vi "Actor Core.vi"(8 "error in":errorcluster, 11 "Sine in":refnum<class "Rigol DG822 Sine.lvclass">) -> (0 "error out":errorcluster, 3 "Actor out":refnum<class "Actor.lvclass">)   [LabVIEW 2021, in "Rigol DG822 UI.lvlib" / "Rigol DG822 Sine.lvlib" / "Rigol DG822 Sine.lvclass"]
uses:
  Rigol DG822 Sine.lvclass
  D:/LabVIEW/General/Files/lvlibp/Actors.lvlibp/Actors/Actors/Actors.lvclass
  General/Files/lvlibp/Actor Framework.lvlibp/1abvi3w/vi.lib/ActorFramework/Actor/Actor.lvclass
  Rigol DG822 UI/lib/controls.llb/WaveformParamTags.ctl
  Rigol DG822 UI/lib/controls.llb/FreqUnitHandler.ctl
  Rigol DG822 UI/lib/controls.llb/DataCluster.ctl
  Rigol DG822 UI/lib/controls.llb/PeriodUnitHandler.ctl
  Rigol DG822 UI/lib/controls.llb/AmplUnitHandler.ctl
  Rigol DG822 UI/lib/controls.llb/HighLUnitHandler.ctl
  Rigol DG822 UI/lib/controls.llb/OffsetUnitHandler.ctl
  Rigol DG822 UI/lib/controls.llb/LowLUnitHandler.ctl
  Rigol DG822 UI/lib/controls.llb/PhaseUnitHandler.ctl
  Rigol DG822 UI/lib/controls.llb/FreqUnit.ctl
  Rigol DG822 UI/lib/controls.llb/PeriodUnit.ctl
  Rigol DG822 UI/lib/controls.llb/AmplUnit.ctl
  Rigol DG822 UI/lib/controls.llb/HighLUnit.ctl
  Rigol DG822 UI/lib/controls.llb/OffsetUnit.ctl
  Rigol DG822 UI/lib/controls.llb/LowLUnit.ctl
  Rigol DG822 UI/lib/controls.llb/SineParamDisplay.ctl
  Rigol DG822 UI/lib/controls.llb/StringIndicatorSelected.ctl
  Rigol DG822 UI/lib/controls.llb/RDG822ExtCall.ctl
  Rigol DG822 UI/lib/controls.llb/FT Controls Cluster.ctl
  Rigol DG822 Sine.lvclass/Rigol DG822 Sine.ctl
  Rigol DG822 UI/lib/controls.llb/WaveformExtCall.ctl
  Rigol DG822 UI/lib/controls.llb/AllWaveformDataCluster.ctl
  Rigol DG822 UI/lib/controls.llb/String Indicators Cluster.ctl
  <vilib>/Utility/miscctls.llb/LVPointTypeDef.ctl
  <userlib>/_MGI/Application Control/MGI VI Reference/MGI Current VI's Reference.vi
  General/Files/lvlibp/Actors.lvlibp/Actors/Actors/Actors.lvclass
panel:
  in  "ParamTags":T1
  out "Data":T2={"Freq"={"Freq"=1.0, "FreqUnit"=enum."kHz", "FreqUnitPrcs"=9.0}, "Period"={"Period"=1.0, "PeriodUnit"=enum."ms", "PeriodUnitPrcs"=7.0}, "Ampl"={"Ampl"=5.0, "AmplUnit"=enum."Vpp", "AmplUnitPrcs"=4.0}, "HighL"={"HighL"=2.5, "HighLUnit"=enum."V", "HighLUnitPrcs"=4.0}, "Offset"={"Offset"=0.0, "OffsetUnit"=enum."Vdc", "OffsetUnitPrcs"=4.0}, "LowL"={"LowL"=-2.5, "LowLUnit"=enum."V", "LowLUnitPrcs"=4.0}, "Phase"={"Phase"=0.0, "PhaseUnit"=enum."°", "PhaseUnitPrcs"=3.0}, "Duty"={"Duty"=50.0, "DutyUnit"=enum."%", "DutyUnitPrcs"=3.0}, "Width"={"Width"=500.0, "WidthUnit"=enum."us", "WidthUnitPrcs"=4.0}, "RisEdge"={"RisEdge"=10.0, "RisEdgeUnit"=enum."ns", "RisEdgeUnitPrcs"=1.0}, "FallEdge"={"FallEdge"=10.0, "FallEdgeUnit"=enum."ns", "FallEdgeUnitPrcs"=1.0}} {"RisEdge"."RisEdge" format="%.1f"; "RisEdge"."RisEdgeUnitPrcs" format="%#_1g"; "FallEdge"."FallEdge" format="%.1f"; "FallEdge"."FallEdgeUnitPrcs" format="%#_1g"; "Width"."Width" format="%.4g"; "Width"."WidthUnitPrcs" format="%#_1g"; "Duty"."Duty" format="%.3g"; "Duty"."DutyUnitPrcs" format="%#_1g"; "Phase"."Phase" format="%.3g"; "Phase"."PhaseUnitPrcs" format="%#_1g"; "LowL"."LowL" format="%.4g"; "LowL"."LowLUnitPrcs" format="%#_1g"; "Offset"."Offset" format="%.4g"; "Offset"."OffsetUnitPrcs" format="%#_1g"; "HighL"."HighL" format="%.4g"; "HighL"."HighLUnitPrcs" format="%#_1g"; "Ampl"."Ampl" format="%.4g"; "Ampl"."AmplUnitPrcs" format="%#_1g"; "Period"."Period" format="%.7g"; "Period"."PeriodUnitPrcs" format="%#_1g"; "Freq"."FreqUnitPrcs" format="%#_1g"; "Freq"."Freq" format="%.9g"}
  in  "Conf Tabs":enum32{"Sine", "OK"}(tab)
  out "SineParamDisplay":T3
  out "String Indcs":T4={"Freq-Period"="1.000,000,000 kHz", "Ampl-HighL"="5.000,0 Vpp", "Offset-LowL"="0.000,0 Vdc", "Phase"="0.000 °"}
  in  "F/T Ctrls":T5
  in  "Value":dbl=1.0 format="%.8g"
  in  "Unit Tabs":T6(tab)
  out "FreqUnitHandler":T7=1
  in  "FreqUnit":T8=enum."kHz"
  out "PeriodUnitHandler":T9=1
  in  "PeriodUnit":T10=enum."ms"
  in  "AmplUnit":T11=enum."Vpp"
  out "AmplUnitHandler":T12
  out "HighLUnitHandler":T13
  in  "HighLUnit":T14=enum."V"
  out "OffsetUnitHandler":T15
  in  "OffsetUnit":T16=enum."Vdc"
  out "LowLUnitHandler":T17
  in  "LowLUnit":T18=enum."V"
  out "PhaseUnitHandler":T19
  in  "OK":bool
  # "MHz - 10 \nkHz - 9\nHz - 6\nmHz - 3\nuHz - 0?"
  # "s - 10\nms - 7\nus - 4 \nns - 1?"
  # "All 4 - V - 4\n        mV - 1"
  # "no change"
  # "no change"
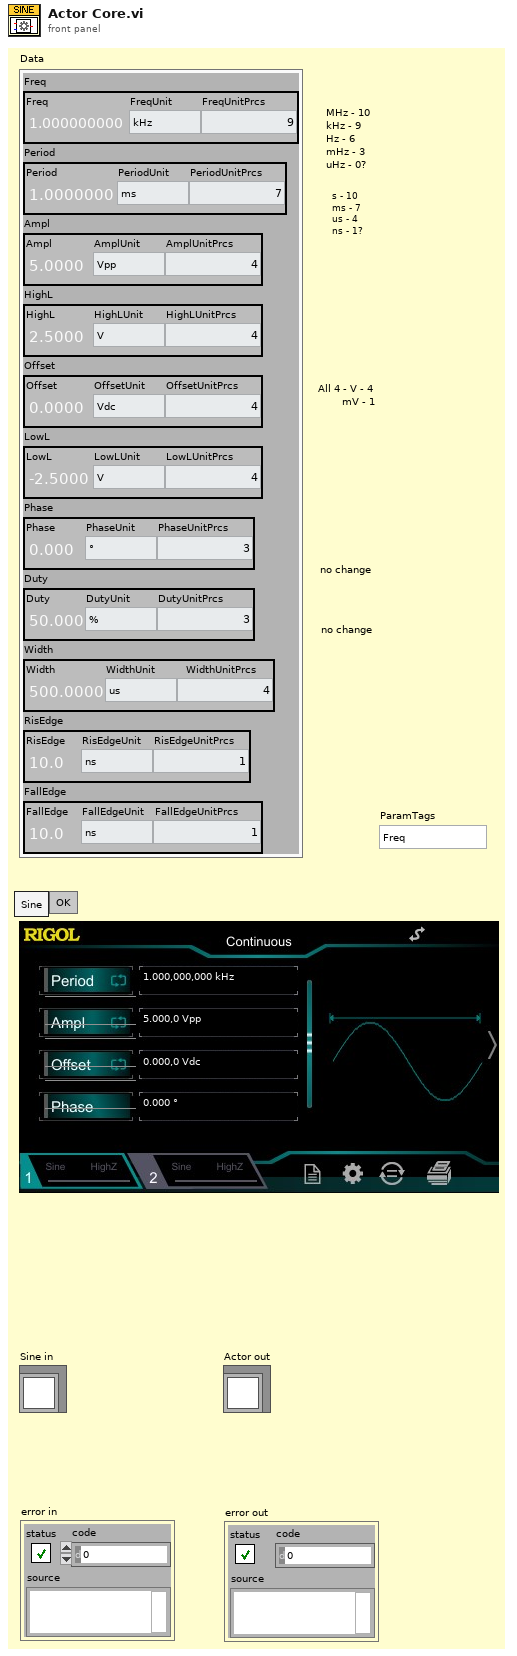
[diagram p1: front panel]
types:
  T1 = typedef "WaveformParamTags.ctl" = enum16{"Freq", "Period", "Ampl", "HighL", "Offset", "LowL", "Phase", "Duty", "Width", "RisEdge", "FallEdge"}
  T2 = typedef "DataCluster.ctl" = cluster{"Freq":cluster{"Freq":dbl, "FreqUnit":enum32{"No Selection", "MHz", "kHz", "Hz", "mHz", "uHz"}, "FreqUnitPrcs":dbl}, "Period":cluster{"Period":dbl, "PeriodUnit":enum32{"No Selection", "s", "ms", "us", "ns"}, "PeriodUnitPrcs":dbl}, "Ampl":cluster{"Ampl":dbl, "AmplUnit":enum32{"No Selection", "Vpp", "mVpp"}, "AmplUnitPrcs":dbl}, "HighL":cluster{"HighL":dbl, "HighLUnit":enum32{"No Selection", "V", "mV"}, "HighLUnitPrcs":dbl}, "Offset":cluster{"Offset":dbl, "OffsetUnit":enum32{"No Selection", "Vdc", "mVdc"}, "OffsetUnitPrcs":dbl}, "LowL":cluster{"LowL":dbl, "LowLUnit":enum32{"No Selection", "V", "mV"}, "LowLUnitPrcs":dbl}, "Phase":cluster{"Phase":dbl, "PhaseUnit":enum32{"°"}, "PhaseUnitPrcs":dbl}, "Duty":cluster{"Duty":dbl, "DutyUnit":enum32{"%"}, "DutyUnitPrcs":dbl}, "Width":cluster{"Width":dbl, "WidthUnit":enum32{"No Selection", "s", "ms", "us", "ns"}, "WidthUnitPrcs":dbl}, "RisEdge":cluster{"RisEdge":dbl, "RisEdgeUnit":enum32{"No Selection", "s", "ms", "us", "ns"}, "RisEdgeUnitPrcs":dbl}, "FallEdge":cluster{"FallEdge":dbl, "FallEdgeUnit":enum32{"No Selection", "s", "ms", "us", "ns"}, "FallEdgeUnitPrcs":dbl}}
  T3 = typedef "SineParamDisplay.ctl" = u16
  T4 = cluster{"Freq-Period":string, "Ampl-HighL":string, "Offset-LowL":string, "Phase":string}
  T5 = cluster{"Freq/Period":bool, "Ampl/HighL":bool, "Offset/LowL":bool}
  T6 = enum32{"Freq", "Period", "Ampl", "HighL", "Offset", "LowL", "Phase"}
  T7 = typedef "FreqUnitHandler.ctl" = u16
  T8 = typedef "FreqUnit.ctl" = enum32{"No Selection", "MHz", "kHz", "Hz", "mHz", "uHz"}
  T9 = typedef "PeriodUnitHandler.ctl" = u16
  T10 = typedef "PeriodUnit.ctl" = enum32{"No Selection", "s", "ms", "us", "ns"}
  T11 = typedef "AmplUnit.ctl" = enum32{"No Selection", "Vpp", "mVpp"}
  T12 = typedef "AmplUnitHandler.ctl" = u16
  T13 = typedef "HighLUnitHandler.ctl" = u16
  T14 = typedef "HighLUnit.ctl" = enum32{"No Selection", "V", "mV"}
  T15 = typedef "OffsetUnitHandler.ctl" = u16
  T16 = typedef "OffsetUnit.ctl" = enum32{"No Selection", "Vdc", "mVdc"}
  T17 = typedef "LowLUnitHandler.ctl" = u16
  T18 = typedef "LowLUnit.ctl" = enum32{"No Selection", "V", "mV"}
  T19 = typedef "PhaseUnitHandler.ctl" = u16
  T20 = cluster{"Freq-Period":string, "Freq-Period 2":string, "Freq-Period 3":string, "Freq-Period 4":string}
  T21 = typedef "LVPointTypeDef.ctl" = cluster{"Horizontal":i16, "Vertical":i16}
  T22 = typedef "StringIndicatorSelected.ctl" = enum16{"Freq-Period", "Ampl-HighL", "Offset-LowL", "Phase", "Duty-Width", "RisEdge", "FallEdge"}
  T23 = typedef "FT Controls Cluster.ctl" = cluster{"Freq/Period":bool, "Ampl/HighL":bool, "Offset/LowL":bool, "Duty/Width":bool}
  T24 = typedef "RDG822ExtCall.ctl" = enum16{"Get Data"}
  T25 = typedef "WaveformExtCall.ctl" = enum16{"Freq", "Period", "Ampl", "HighL", "Offset", "LowL", "Phase", "Duty", "Width", "RisEdge", "FallEdge", "Home", "InitData"}
  T26 = cluster{"Freq":cluster{"Freq":dbl, "FreqUnit":enum32{"No Selection", "MHz", "kHz", "Hz", "mHz", "uHz"}, "FreqUnitPrcs":dbl}, "Period":cluster{"Period":dbl, "PeriodUnit":enum32{"No Selection", "s", "ms", "us", "ns"}, "PeriodUnitPrcs":dbl}}
  T27 = cluster{"Ampl":cluster{"Ampl":dbl, "AmplUnit":enum32{"No Selection", "Vpp", "mVpp"}, "AmplUnitPrcs":dbl}, "HighL":cluster{"HighL":dbl, "HighLUnit":enum32{"No Selection", "V", "mV"}, "HighLUnitPrcs":dbl}, "Offset":cluster{"Offset":dbl, "OffsetUnit":enum32{"No Selection", "Vdc", "mVdc"}, "OffsetUnitPrcs":dbl}, "LowL":cluster{"LowL":dbl, "LowLUnit":enum32{"No Selection", "V", "mV"}, "LowLUnitPrcs":dbl}}
  T28 = cluster{"Phase":dbl, "PhaseUnit":enum32{"°"}, "PhaseUnitPrcs":dbl}
  T29 = typedef "AllWaveformDataCluster.ctl" = cluster{"Data":T2, "F/T Ctrls":T23, "String Indcs":T30}
  T30 = typedef "String Indicators Cluster.ctl" = cluster{"Freq-Period":string, "Ampl-HighL":string, "Offset-LowL":string, "Phase":string, "Duty-Width":string, "RisEdge":string, "FallEdge":string}
  T31 = enum32{"No Selection", "MHz", "kHz", "Hz", "mHz", "uHz"}
  T32 = cluster{"Value":dbl, "PeriodUnit":u32, "FreqUnitPrecision":dbl}
  T33 = cluster{"Freq":dbl, "FreqUnit":enum32{"No Selection", "MHz", "kHz", "Hz", "mHz", "uHz"}, "FreqUnitPrcs":dbl}
  T34 = cluster{"Period":dbl, "PeriodUnit":enum32{"No Selection", "s", "ms", "us", "ns"}, "PeriodUnitPrcs":dbl}
  T35 = cluster{"Ampl":dbl, "AmplUnit":enum32{"No Selection", "Vpp", "mVpp"}, "AmplUnitPrcs":dbl}
  T36 = cluster{"HighL":dbl, "HighLUnit":enum32{"No Selection", "V", "mV"}, "HighLUnitPrcs":dbl}
  T37 = cluster{"Offset":dbl, "OffsetUnit":enum32{"No Selection", "Vdc", "mVdc"}, "OffsetUnitPrcs":dbl}
  T38 = cluster{"LowL":dbl, "LowLUnit":enum32{"No Selection", "V", "mV"}, "LowLUnitPrcs":dbl}
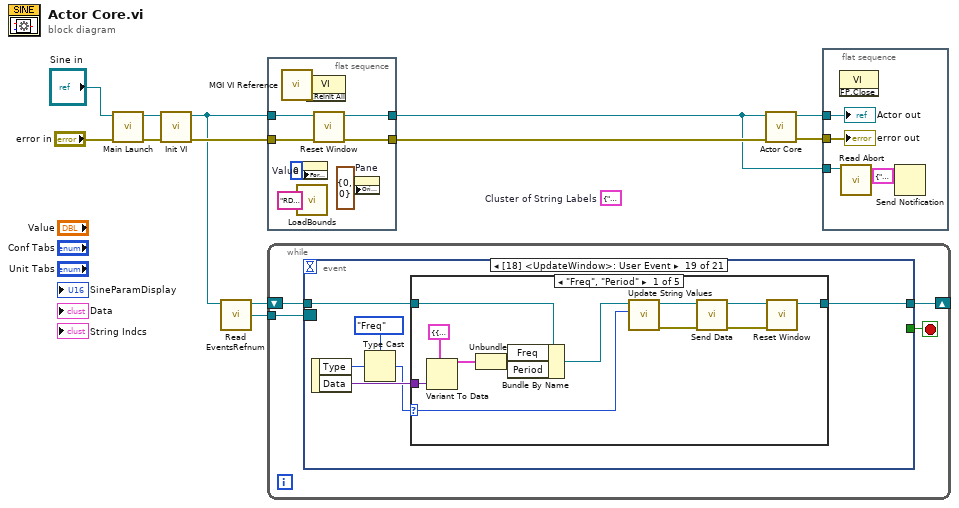
[diagram p0: block diagram]
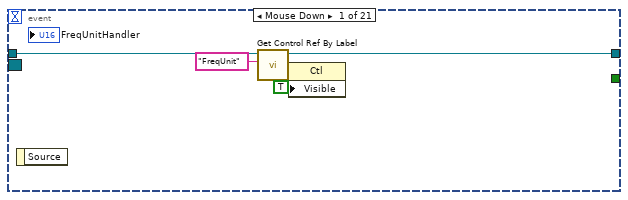
[diagram p2: hidden frame]
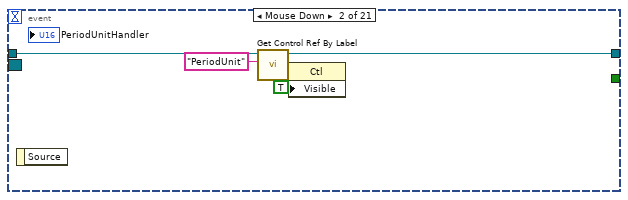
[diagram p3: hidden frame]
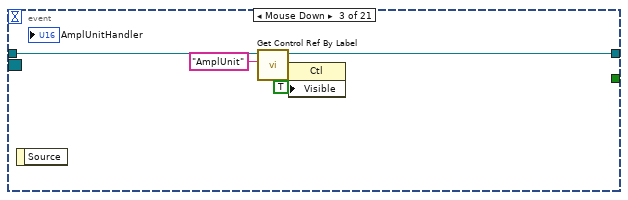
[diagram p4: hidden frame]
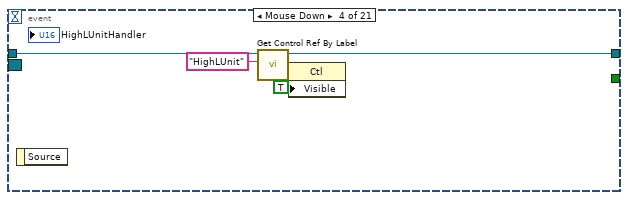
[diagram p5: hidden frame]
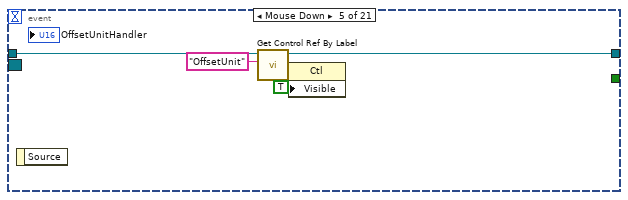
[diagram p6: hidden frame]
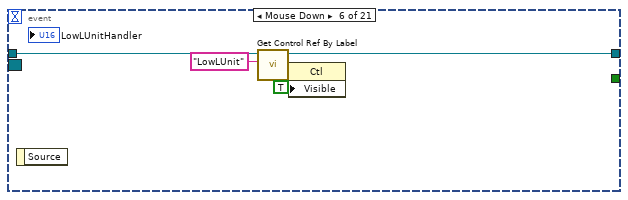
[diagram p7: hidden frame]
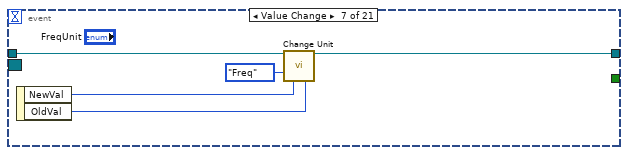
[diagram p8: hidden frame]
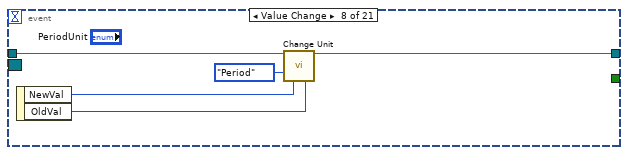
[diagram p9: hidden frame]
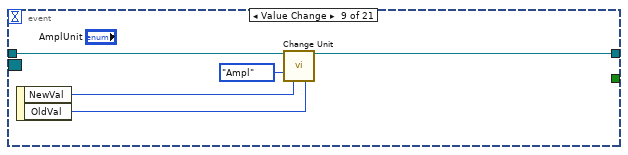
[diagram p10: hidden frame]
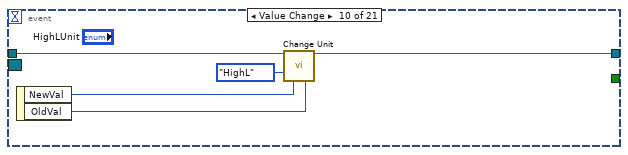
[diagram p11: hidden frame]
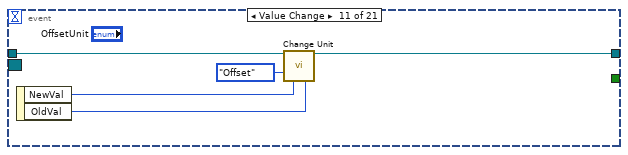
[diagram p12: hidden frame]
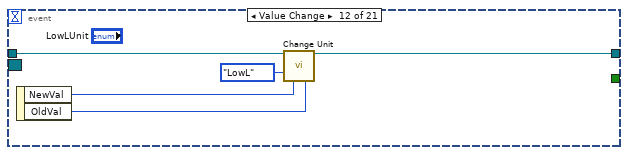
[diagram p13: hidden frame]
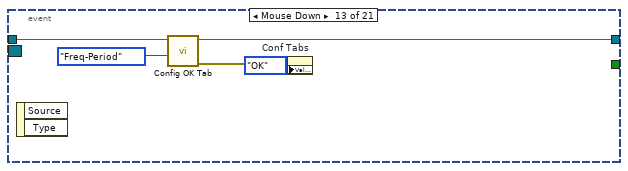
[diagram p14: hidden frame]
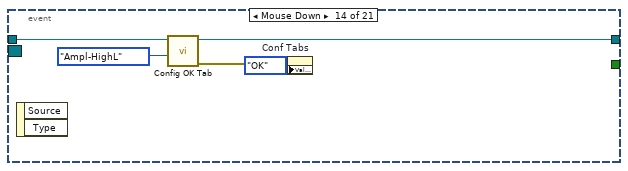
[diagram p15: hidden frame]
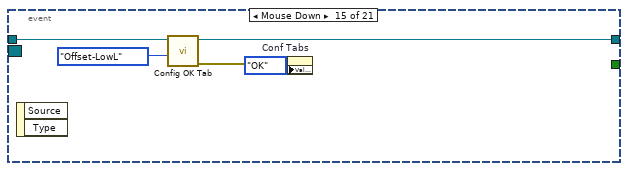
[diagram p16: hidden frame]
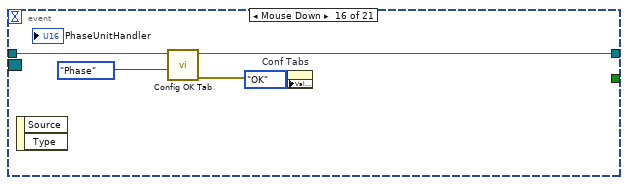
[diagram p17: hidden frame]
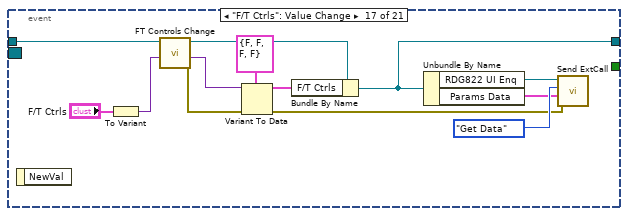
[diagram p18: hidden frame]
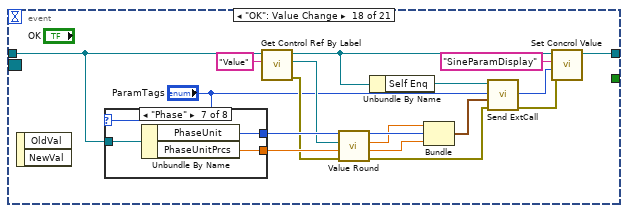
[diagram p19: hidden frame]
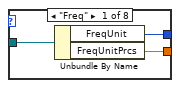
[diagram p20: hidden frame]
diagram:
  (unwired) T20 {"Freq-Period"="String Indcs.Freq-Period", "Freq-Period 2"="String Indcs.Ampl-HighL", "Freq-Period 3"="String Indcs.Offset-LowL", "Freq-Period 4"="String Indcs.Phase"}  # Cluster of String Labels
  n1 = call "Main Launch.vi"("error in (no error)"="error in", "Actors in"="Sine in") -> ("error out"=w3:errorcluster, "Actors out"=w2:refnum<class "Rigol DG822 Sine.lvclass">)  [unwired: 6 in, 2 out]
  n2 = call-dynamic "Init VI.vi"("error in (no error)"=w3, "Rigol DG822 Sine in"=w2) -> ("error out"=w4:errorcluster, "Rigol DG822 Sine out"=w1:refnum<class "Rigol DG822 Sine.lvclass">)  [unwired: 8 in]
  n3 = call "Read EventsRefnum.vi"("Actors in"=w1) -> ("EventsRefnum"=w7:refnum<event-registration>, "Actors out"=w6:refnum<class "Rigol DG822 Sine.lvclass">)  [unwired: 9 in]
  n4 = flat-sequence {
    tunnel: w4 -> [w14]
    tunnel: [w17] -> w10
    tunnel: w1 -> [w15]
    tunnel: [w16] -> w5
    frame #0 {
      n5 = call-poly <userlib>:"MGI VI Reference.vi"() -> ("Current VI's Reference"=w13:refnum<vi>)  [unwired: 1 in]
      n6 = call "LoadBounds.vi"("SettingName"="RDG822Sine.bounds") -> ()
      n7 = property on="Value" class="DigNum (strict)"("Format"=u8 0 ("Display Format:Format")) -> ()  [unwired: 2 in, 2 out]
      n8 = invoke class="VI" method="Default Vals.Reinit All"(reference=w13) -> ()  [unwired: 2 in, 3 out]
      n9 = call-dynamic "Reset Window.vi"("error in (no error)"=w14, "Rigol DG822 Sine in"=w15) -> ("error out"=w17:errorcluster, "Rigol DG822 Sine out"=w16:refnum<class "Rigol DG822 Sine.lvclass">)  [unwired: 8 in]
      n10 = property on="Pane" class="Pane"("Origin"=T21 {"Horizontal"=0, "Vertical"=0}) -> ()  [unwired: 2 in, 2 out]
    }
  }
  n11 = while {
    tunnel: w7 -> [w24]
    shift-right: [w22] -> _
    shift-left: w6 -> [w23]
    stop <- w21 stop-if-true
    n12 = event shown="[18] <UpdateWindow>: User Event" {
      selector: w24 -> [_ _ _ _ _ _ _ _ _ _ _ _ _ _ _ _ _ _ _ _ w233]
      dyn-events: _ -> [_ _ _ _ _ _ _ _ _ _ _ _ _ _ _ _ _ _ _ _ _]
      timeout: _ -> [_ _ _ _ _ _ _ _ _ _ _ _ _ _ _ _ _ _ _ _ _]
      tunnel: w23 -> [w30 w36 w42 w48 w54 w60 w65 w70 w75 w80 w85 w90 w93 w98 w103 w108 w123 w134 w166 w221 w231]
      tunnel: [w29 w35 w41 w47 w53 w59 w64 w69 w74 w79 w84 w89 w94 w99 w104 w109 w115 w128 w167 w218 w229] -> w22
      tunnel: [_ _ _ _ _ _ _ _ _ _ _ _ _ _ _ _ _ _ _ _ w234] -> w21
      event Mouse Down {
        n13 = event-data() -> ()  [unwired: 1 in, 1 out]
        n14 = call "Get Control Ref By Label.vi"("Control Label"="FreqUnit", "Actors in"=w30) -> ("error out"=w25:errorcluster, "Control Ref"=w27:refnum<vi>, "Actors out"=w29:refnum<class "Rigol DG822 Sine.lvclass">)  [unwired: 7 in]
        n15 = property class="Ctl"(reference=w27, error in=w25, "Visible"=TRUE) -> ()  [unwired: 2 out]
      }
      event Mouse Down {
        n16 = event-data() -> ()  [unwired: 1 in, 1 out]
        n17 = call "Get Control Ref By Label.vi"("Control Label"="PeriodUnit", "Actors in"=w36) -> ("error out"=w31:errorcluster, "Control Ref"=w33:refnum<vi>, "Actors out"=w35:refnum<class "Rigol DG822 Sine.lvclass">)  [unwired: 7 in]
        n18 = property class="Ctl"(reference=w33, error in=w31, "Visible"=TRUE) -> ()  [unwired: 2 out]
      }
      event Mouse Down {
        n19 = event-data() -> ()  [unwired: 1 in, 1 out]
        n20 = call "Get Control Ref By Label.vi"("Control Label"="AmplUnit", "Actors in"=w42) -> ("error out"=w37:errorcluster, "Control Ref"=w39:refnum<vi>, "Actors out"=w41:refnum<class "Rigol DG822 Sine.lvclass">)  [unwired: 7 in]
        n21 = property class="Ctl"(reference=w39, error in=w37, "Visible"=TRUE) -> ()  [unwired: 2 out]
      }
      event Mouse Down {
        n22 = event-data() -> ()  [unwired: 1 in, 1 out]
        n23 = call "Get Control Ref By Label.vi"("Control Label"="HighLUnit", "Actors in"=w48) -> ("error out"=w43:errorcluster, "Control Ref"=w45:refnum<vi>, "Actors out"=w47:refnum<class "Rigol DG822 Sine.lvclass">)  [unwired: 7 in]
        n24 = property class="Ctl"(reference=w45, error in=w43, "Visible"=TRUE) -> ()  [unwired: 2 out]
      }
      event Mouse Down {
        n25 = event-data() -> ()  [unwired: 1 in, 1 out]
        n26 = call "Get Control Ref By Label.vi"("Control Label"="OffsetUnit", "Actors in"=w54) -> ("error out"=w49:errorcluster, "Control Ref"=w51:refnum<vi>, "Actors out"=w53:refnum<class "Rigol DG822 Sine.lvclass">)  [unwired: 7 in]
        n27 = property class="Ctl"(reference=w51, error in=w49, "Visible"=TRUE) -> ()  [unwired: 2 out]
      }
      event Mouse Down {
        n28 = event-data() -> ()  [unwired: 1 in, 1 out]
        n29 = call "Get Control Ref By Label.vi"("Control Label"="LowLUnit", "Actors in"=w60) -> ("error out"=w55:errorcluster, "Control Ref"=w57:refnum<vi>, "Actors out"=w59:refnum<class "Rigol DG822 Sine.lvclass">)  [unwired: 7 in]
        n30 = property class="Ctl"(reference=w57, error in=w55, "Visible"=TRUE) -> ()  [unwired: 2 out]
      }
      event Value Change {
        n31 = event-data() -> ("NewVal"=w63:T8, "OldVal"=w62:T8)  [unwired: 1 in]
        n32 = call-dynamic "Change Unit.vi"("Rigol DG822 Sine in"=w65, "ParamTags"=WaveformParamTags."Freq", "New Value"=w63, "Old Value"=w62) -> ("Rigol DG822 Sine out"=w64:refnum<class "Rigol DG822 Sine.lvclass">)  [unwired: 10 in, 1 out]
      }
      event Value Change {
        n33 = event-data() -> ("NewVal"=w68:T10, "OldVal"=w67:T10)  [unwired: 1 in]
        n34 = call-dynamic "Change Unit.vi"("Rigol DG822 Sine in"=w70, "ParamTags"=WaveformParamTags."Period", "New Value"=w68, "Old Value"=w67) -> ("Rigol DG822 Sine out"=w69:refnum<class "Rigol DG822 Sine.lvclass">)  [unwired: 10 in, 1 out]
      }
      event Value Change {
        n35 = event-data() -> ("NewVal"=w73:T11, "OldVal"=w72:T11)  [unwired: 1 in]
        n36 = call-dynamic "Change Unit.vi"("Rigol DG822 Sine in"=w75, "ParamTags"=WaveformParamTags."Ampl", "New Value"=w73, "Old Value"=w72) -> ("Rigol DG822 Sine out"=w74:refnum<class "Rigol DG822 Sine.lvclass">)  [unwired: 10 in, 1 out]
      }
      event Value Change {
        n37 = event-data() -> ("NewVal"=w78:T14, "OldVal"=w77:T14)  [unwired: 1 in]
        n38 = call-dynamic "Change Unit.vi"("Rigol DG822 Sine in"=w80, "ParamTags"=WaveformParamTags."HighL", "New Value"=w78, "Old Value"=w77) -> ("Rigol DG822 Sine out"=w79:refnum<class "Rigol DG822 Sine.lvclass">)  [unwired: 10 in, 1 out]
      }
      event Value Change {
        n39 = event-data() -> ("NewVal"=w83:T16, "OldVal"=w82:T16)  [unwired: 1 in]
        n40 = call-dynamic "Change Unit.vi"("Rigol DG822 Sine in"=w85, "ParamTags"=WaveformParamTags."Offset", "New Value"=w83, "Old Value"=w82) -> ("Rigol DG822 Sine out"=w84:refnum<class "Rigol DG822 Sine.lvclass">)  [unwired: 10 in, 1 out]
      }
      event Value Change {
        n41 = event-data() -> ("NewVal"=w88:T18, "OldVal"=w87:T18)  [unwired: 1 in]
        n42 = call-dynamic "Change Unit.vi"("Rigol DG822 Sine in"=w90, "ParamTags"=WaveformParamTags."LowL", "New Value"=w88, "Old Value"=w87) -> ("Rigol DG822 Sine out"=w89:refnum<class "Rigol DG822 Sine.lvclass">)  [unwired: 10 in, 1 out]
      }
      event "String Indcs.Freq-Period": Mouse Down {
        n43 = event-data() -> ()  [unwired: 1 in, 2 out]
        n44 = call-dynamic "Config OK Tab.vi"("String Selected"=StringIndicatorSelected."Freq-Period", "Rigol DG822 Sine in"=w93) -> ("error out"=w92:errorcluster, "Rigol DG822 Sine out"=w94:refnum<class "Rigol DG822 Sine.lvclass">)  [unwired: 8 in]
        n45 = property on="Conf Tabs" class="TabCtl (strict)"(error in=w92, "Value"=enum32{"Sine", "OK"}."OK" ("Sine Tabs")) -> ()  [unwired: 1 in, 2 out]
      }
      event "String Indcs.Ampl-HighL": Mouse Down {
        n46 = event-data() -> ()  [unwired: 1 in, 2 out]
        n47 = call-dynamic "Config OK Tab.vi"("String Selected"=StringIndicatorSelected."Ampl-HighL", "Rigol DG822 Sine in"=w98) -> ("error out"=w97:errorcluster, "Rigol DG822 Sine out"=w99:refnum<class "Rigol DG822 Sine.lvclass">)  [unwired: 8 in]
        n48 = property on="Conf Tabs" class="TabCtl (strict)"(error in=w97, "Value"=enum32{"Sine", "OK"}."OK" ("Sine Tabs")) -> ()  [unwired: 1 in, 2 out]
      }
      event "String Indcs.Offset-LowL": Mouse Down {
        n49 = event-data() -> ()  [unwired: 1 in, 2 out]
        n50 = call-dynamic "Config OK Tab.vi"("String Selected"=StringIndicatorSelected."Offset-LowL", "Rigol DG822 Sine in"=w103) -> ("error out"=w102:errorcluster, "Rigol DG822 Sine out"=w104:refnum<class "Rigol DG822 Sine.lvclass">)  [unwired: 8 in]
        n51 = property on="Conf Tabs" class="TabCtl (strict)"(error in=w102, "Value"=enum32{"Sine", "OK"}."OK" ("Sine Tabs")) -> ()  [unwired: 1 in, 2 out]
      }
      event "String Indcs.Phase": Mouse Down {
        n52 = event-data() -> ()  [unwired: 1 in, 2 out]
        n53 = call-dynamic "Config OK Tab.vi"("String Selected"=StringIndicatorSelected."Phase", "Rigol DG822 Sine in"=w108) -> ("error out"=w107:errorcluster, "Rigol DG822 Sine out"=w109:refnum<class "Rigol DG822 Sine.lvclass">)  [unwired: 8 in]
        n54 = property on="Conf Tabs" class="TabCtl (strict)"(error in=w107, "Value"=enum32{"Sine", "OK"}."OK" ("Sine Tabs")) -> ()  [unwired: 1 in, 2 out]
      }
      event "F/T Ctrls": Value Change {
        n55 = event-data() -> ()  [unwired: 1 in, 1 out]
        n56 = To Variant(anything="F/T Ctrls") -> (Variant=w121:variant)
        n57 = call-dynamic "FT Controls Change.vi"("F/T Ctrls Cluster Variant"=w121, "Rigol DG822 Sine in"=w123) -> ("error out"=w113:errorcluster, "New F/T Ctrls Cluster Variant"=w120:variant, "Rigol DG822 Sine out"=w122:refnum<class "Rigol DG822 Sine.lvclass">)  [unwired: 7 in]
        n58 = Variant To Data(error in=w113, type=T23 {"Freq/Period"=FALSE, "Ampl/HighL"=FALSE, "Offset/LowL"=FALSE, "Duty/Width"=FALSE} ("F/T Ctrls"), Variant=w120) -> (data=w119:T23, error out=w112:errorcluster)
        n59 = Bundle By Name(cluster=w122, "F/T Ctrls"=w119) -> (w115:refnum<class "Rigol DG822 Sine.lvclass">)
        n60 = Unbundle By Name(w115) -> ("RDG822 UI Enq"=w118:refnum<class "Message Enqueuer.lvclass">, "Params Data"=w116:T29)
        n61 = call "Send ExtCall.vi"("error in (no error)"=w112, "Val"=w116, "Tag"=RDG822ExtCall."Get Data", "Message Enqueuer"=w118) -> ()  [unwired: 4 in, 4 out]
      }
      event "OK": Value Change {
        n62 = event-data() -> ()  [unwired: 1 in, 2 out]
        n63 = case shown="\"Phase\"" "ParamTags" {
          tunnel: [w139 w142 w145 w148 w151 w154 w157 4.0 ("FreqUnitPrecision")] -> w135
          tunnel: [w141 w144 w147 w150 w153 w156 w159 1] -> w136
          tunnel: w134 -> [w140 w143 w146 w149 w152 w155 w158 _]
          frame "Freq" {
            n64 = Unbundle By Name(w140) -> ("FreqUnit"=w141:T31, "FreqUnitPrcs"=w139:dbl)
          }
          frame "Period" {
            n65 = Unbundle By Name(w143) -> ("PeriodUnit"=w144:enum32{"No Selection", "s", "ms", "us", "ns"}, "PeriodUnitPrcs"=w142:dbl)
          }
          frame "Ampl" {
            n66 = Unbundle By Name(w146) -> ("AmplUnit"=w147:enum32{"No Selection", "Vpp", "mVpp"}, "AmplUnitPrcs"=w145:dbl)
          }
          frame "HighL" {
            n67 = Unbundle By Name(w149) -> ("HighLUnit"=w150:enum32{"No Selection", "V", "mV"}, "HighLUnitPrcs"=w148:dbl)
          }
          frame "Offset" {
            n68 = Unbundle By Name(w152) -> ("OffsetUnit"=w153:enum32{"No Selection", "Vdc", "mVdc"}, "OffsetUnitPrcs"=w151:dbl)
          }
          frame "LowL" {
            n69 = Unbundle By Name(w155) -> ("LowLUnit"=w156:enum32{"No Selection", "V", "mV"}, "LowLUnitPrcs"=w154:dbl)
          }
          frame "Phase" {
            n70 = Unbundle By Name(w158) -> ("PhaseUnit"=w159:enum32{"°"}, "PhaseUnitPrcs"=w157:dbl)
          }
          frame Default {
          }
        }
        n71 = call "Get Control Ref By Label.vi"("Control Label"="Value", "Actors in"=w134) -> ("error out"=w131:errorcluster, "Control Ref"=w133:refnum<vi>, "Actors out"=w127:refnum<class "Rigol DG822 Sine.lvclass">)  [unwired: 7 in]
        n72 = call "Value Round.vi"("error in (no error)"=w131, "UnitPrecision"=w135, "Value Ref"=w133) -> ("error out"=w130:errorcluster, "Value"=w129:dbl)  [unwired: 7 in]
        n73 = Unbundle By Name(w127) -> ("Self Enq"=w138:refnum<class "Message Enqueuer.lvclass">)
        n74 = Bundle("Value"=w129, "PeriodUnit"=w136, "FreqUnitPrecision"=w135) -> (w137:T32)  [unwired: 1 in]
        n75 = call "Send ExtCall.vi"("error in (no error)"=w130, "Val"=w137, "Tag"="ParamTags", "Message Enqueuer"=w138) -> ("error out"=w124:errorcluster)  [unwired: 4 in, 3 out]
        n76 = call "Set Concrol Value.vi"("error in (no error)"=w124, "Value"="ParamTags", "Control Label"="SineParamDisplay", "Actors in"=w127) -> ("Actors out"=w128:refnum<class "Rigol DG822 Sine.lvclass">)  [unwired: 6 in, 1 out]
      }
      event User Event {
        n77 = event-data() -> ("Type"=w164:u16, "Data"=w165:variant)  [unwired: 1 in]
        n78 = Type Cast(type=WaveformExtCall."Freq" ("Enum"), x=w164) -> (*(type *) &x=w163:T25)
        n79 = case shown="\"Freq\", \"Period\"" w163 {
          selector: w163 -> [w178 w194 w205 _ _]
          tunnel: [w176 w193 w204 w208 w215] -> w167
          tunnel: w166 -> [w179 w186 w203 w209 w217]
          tunnel: w165 -> [w180 w195 w206 _ w216]
          frame "Freq", "Period" {
            n80 = Variant To Data(type=T26 {"Freq"={"Freq"=1.0, "FreqUnit"=enum."kHz", "FreqUnitPrcs"=9.0}, "Period"={"Period"=1.0, "PeriodUnit"=enum."ms", "PeriodUnitPrcs"=7.0}}, Variant=w180) -> (data=w175:T26)  [unwired: 1 in, 1 out]
            n81 = Unbundle(w175) -> ("Freq"=w174:T33, "Period"=w173:T34)
            n82 = Bundle By Name(cluster=w179, "Freq"=w174, "Period"=w173) -> (w177:refnum<class "Rigol DG822 Sine.lvclass">)
            n83 = call-dynamic "Update String Values.vi"("Type"=w178, "Rigol DG822 Sine in"=w177) -> ("error out"=w169:errorcluster, "Rigol DG822 Sine out"=w171:refnum<class "Rigol DG822 Sine.lvclass">)  [unwired: 8 in]
            n84 = call-dynamic "Send Data.vi"("error in (no error)"=w169, "Rigol DG822 Sine in"=w171) -> ("error out"=w168:errorcluster, "Rigol DG822 Sine out"=w170:refnum<class "Rigol DG822 Sine.lvclass">)  [unwired: 8 in]
            n85 = call-dynamic "Reset Window.vi"("error in (no error)"=w168, "Rigol DG822 Sine in"=w170) -> ("Rigol DG822 Sine out"=w176:refnum<class "Rigol DG822 Sine.lvclass">)  [unwired: 8 in, 1 out]
          }
          frame "Ampl".."LowL" {
            n86 = Variant To Data(type=T27 {"Ampl"={"Ampl"=5.0, "AmplUnit"=enum."Vpp", "AmplUnitPrcs"=4.0}, "HighL"={"HighL"=2.5, "HighLUnit"=enum."V", "HighLUnitPrcs"=4.0}, "Offset"={"Offset"=0.0, "OffsetUnit"=enum."Vdc", "OffsetUnitPrcs"=4.0}, "LowL"={"LowL"=-2.5, "LowLUnit"=enum."V", "LowLUnitPrcs"=4.0}}, Variant=w195) -> (data=w192:T27)  [unwired: 1 in, 1 out]
            n87 = Unbundle(w192) -> ("Ampl"=w190:T35, "HighL"=w187:T36, "Offset"=w188:T37, "LowL"=w189:T38)
            n88 = Bundle By Name(cluster=w186, "Ampl"=w190, "HighL"=w187, "Offset"=w188, "LowL"=w189) -> (w185:refnum<class "Rigol DG822 Sine.lvclass">)
            n89 = call-dynamic "Update String Values.vi"("Type"=w194, "Rigol DG822 Sine in"=w185) -> ("error out"=w183:errorcluster, "Rigol DG822 Sine out"=w184:refnum<class "Rigol DG822 Sine.lvclass">)  [unwired: 8 in]
            n90 = call-dynamic "Send Data.vi"("error in (no error)"=w183, "Rigol DG822 Sine in"=w184) -> ("error out"=w181:errorcluster, "Rigol DG822 Sine out"=w182:refnum<class "Rigol DG822 Sine.lvclass">)  [unwired: 8 in]
            n91 = call-dynamic "Reset Window.vi"("error in (no error)"=w181, "Rigol DG822 Sine in"=w182) -> ("Rigol DG822 Sine out"=w193:refnum<class "Rigol DG822 Sine.lvclass">)  [unwired: 8 in, 1 out]
          }
          frame "Phase" {
            n92 = Variant To Data(type=T28 {"Phase"=0.0, "PhaseUnit"=enum."°", "PhaseUnitPrcs"=3.0} ("Phase"), Variant=w206) -> (data=w201:T28)  [unwired: 1 in, 1 out]
            n93 = Bundle By Name(cluster=w203, "Phase"=w201) -> (w202:refnum<class "Rigol DG822 Sine.lvclass">)
            n94 = call-dynamic "Update String Values.vi"("Type"=w205, "Rigol DG822 Sine in"=w202) -> ("error out"=w198:errorcluster, "Rigol DG822 Sine out"=w199:refnum<class "Rigol DG822 Sine.lvclass">)  [unwired: 8 in]
            n95 = call-dynamic "Send Data.vi"("error in (no error)"=w198, "Rigol DG822 Sine in"=w199) -> ("error out"=w197:errorcluster, "Rigol DG822 Sine out"=w196:refnum<class "Rigol DG822 Sine.lvclass">)  [unwired: 8 in]
            n96 = call-dynamic "Reset Window.vi"("error in (no error)"=w197, "Rigol DG822 Sine in"=w196) -> ("Rigol DG822 Sine out"=w204:refnum<class "Rigol DG822 Sine.lvclass">)  [unwired: 8 in, 1 out]
          }
          frame "Home", Default {
            n97 = property on="Conf Tabs" class="TabCtl (strict)"("Value"=enum32{"Sine", "OK"}."Sine" ("Sine Tabs")) -> (error out=w207:errorcluster)  [unwired: 2 in, 1 out]
            n98 = call-dynamic "Reset Window.vi"("error in (no error)"=w207, "Rigol DG822 Sine in"=w209) -> ("Rigol DG822 Sine out"=w208:refnum<class "Rigol DG822 Sine.lvclass">)  [unwired: 8 in, 1 out]
          }
          frame "InitData" {
            n99 = Variant To Data(type=T29 {"Data"={"Freq"={"Freq"=1.0, "FreqUnit"=enum."kHz", "FreqUnitPrcs"=9.0}, "Period"={"Period"=1.0, "PeriodUnit"=enum."ms", "PeriodUnitPrcs"=7.0}, "Ampl"={"Ampl"=5.0, "AmplUnit"=enum."Vpp", "AmplUnitPrcs"=4.0}, "HighL"={"HighL"=2.5, "HighLUnit"=enum."V", "HighLUnitPrcs"=4.0}, "Offset"={"Offset"=0.0, "OffsetUnit"=enum."Vdc", "OffsetUnitPrcs"=4.0}, "LowL"={"LowL"=-2.5, "LowLUnit"=enum."V", "LowLUnitPrcs"=4.0}, "Phase"={"Phase"=0.0, "PhaseUnit"=enum."°", "PhaseUnitPrcs"=3.0}, "Duty"={"Duty"=50.0, "DutyUnit"=enum."%", "DutyUnitPrcs"=3.0}, "Width"={"Width"=500.0, "WidthUnit"=enum."us", "WidthUnitPrcs"=4.0}, "RisEdge"={"RisEdge"=10.0, "RisEdgeUnit"=enum."ns", "RisEdgeUnitPrcs"=1.0}, "FallEdge"={"FallEdge"=10.0, "FallEdgeUnit"=enum."ns", "FallEdgeUnitPrcs"=1.0}}, "F/T Ctrls"={"Freq/Period"=FALSE, "Ampl/HighL"=FALSE, "Offset/LowL"=FALSE, "Duty/Width"=FALSE}, "String Indcs"={"Freq-Period"="1.000,000,000 kHz", "Ampl-HighL"="5.000,0 Vpp", "Offset-LowL"="0.000,0 Vdc", "Phase"="0.000 °", "Duty-Width"="50.000 %", "RisEdge"="10.0 ns", "FallEdge"="10.0 ns"}} ("Params Data"), Variant=w216) -> (data=w213:T29, error out=w211:errorcluster)  [unwired: 1 in]
            n100 = Bundle By Name(cluster=w217, "Params Data"=w213) -> (w214:refnum<class "Rigol DG822 Sine.lvclass">)
            n101 = call-dynamic "Init Data.vi"("error in (no error)"=w211, "Rigol DG822 Sine in"=w214) -> ("Rigol DG822 Sine out"=w215:refnum<class "Rigol DG822 Sine.lvclass">)  [unwired: 8 in, 1 out]
          }
        }
      }
      event Panel Close? {
        n102 = event-data() -> ()  [unwired: 1 in, 1 out]
        n103 = flat-sequence {
          tunnel: w221 -> [w224]
          tunnel: [w224] -> w220
          tunnel: w220 -> [w226]
          tunnel: [w225] -> w219
          tunnel: [TRUE] -> w222
          tunnel: [w227] -> w218
          tunnel: w219 -> [w227]
          frame #0 {
            n104 = call "SaveBounds.vi"("SettingName"="RDG822Sine.bounds") -> ()
          }
          frame #1 {
            n105 = call "SetClose.vi"("Actors in"=w226) -> ("Actors out"=w225:refnum<class "Rigol DG822 Sine.lvclass">)  [unwired: 9 in, 1 out]
          }
          frame #2 {
          }
        }
        n106 = event-data("Discard?"=w222) -> ()  [unwired: 1 in, 1 out]
      }
      event User Event {
        n107 = event-data() -> ()  [unwired: 1 in, 1 out]
        n108 = flat-sequence {
          tunnel: w233 -> [w236]
          tunnel: [w235] -> w232
          tunnel: w231 -> [w235]
          tunnel: w232 -> [w237]
          tunnel: [w237] -> w230
          tunnel: [TRUE] -> w234
          tunnel: w230 -> [w238]
          tunnel: [w238] -> w229
          frame #0 {
            n109 = Unregister For Events(event registration refnum=w236) -> ()  [unwired: 1 in, 1 out]
          }
          frame #1 {
          }
          frame #2 {
          }
        }
      }
    }
  }
  n110 = call-parent "Actor Core.vi"("error in"=w10, "Actor in"=w5) -> ("error out"=w8:errorcluster, "Actor out"=w9:refnum<class "Actor.lvclass">)  [unwired: 8 in]
  n111 = flat-sequence {
    tunnel: w9 -> [w244]
    tunnel: w8 -> [w243]
    tunnel: w5 -> [w240]
    frame #0 {
      n112 = invoke class="VI" method="FP.Close"() -> ()  [unwired: 3 in, 3 out]
      n113 = call "Read Abort.vi"("Actors in"=w240) -> ("AbortEvent"=w242:refnum<notifier>)  [unwired: 10 in]
      n114 = Send Notification(notification=cluster{"Caller":string, "AnyValue":variant} {"Caller"="abort", "AnyValue"=variant}, notifier=w242) -> ()  [unwired: 1 in, 2 out]
      "Actor out" <- w244
      "error out" <- w243
    }
  }
